vi "createPattern.vi"(7 "Numeric":i32=50, 11 "Refnum in":T1) -> (3 "Image Out 3":T1)   [LabVIEW 2020]
uses:
  <vilib>/vision/Image Controls.llb/IMAQ Image.ctl
  <vilib>/Analysis/1siggen.llb/Ramp Pattern by Samples.vi
  <vilib>/vision/NI_Vision_Development_Module.lvlib
  <vilib>/Analysis/NI_AALBase.lvlib
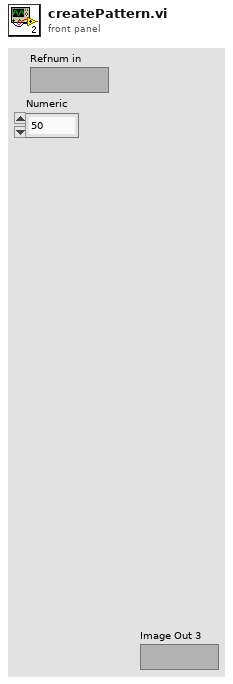
[diagram p1: front panel]
types:
  T1 = typedef "IMAQ Image.ctl" = refnum<image>
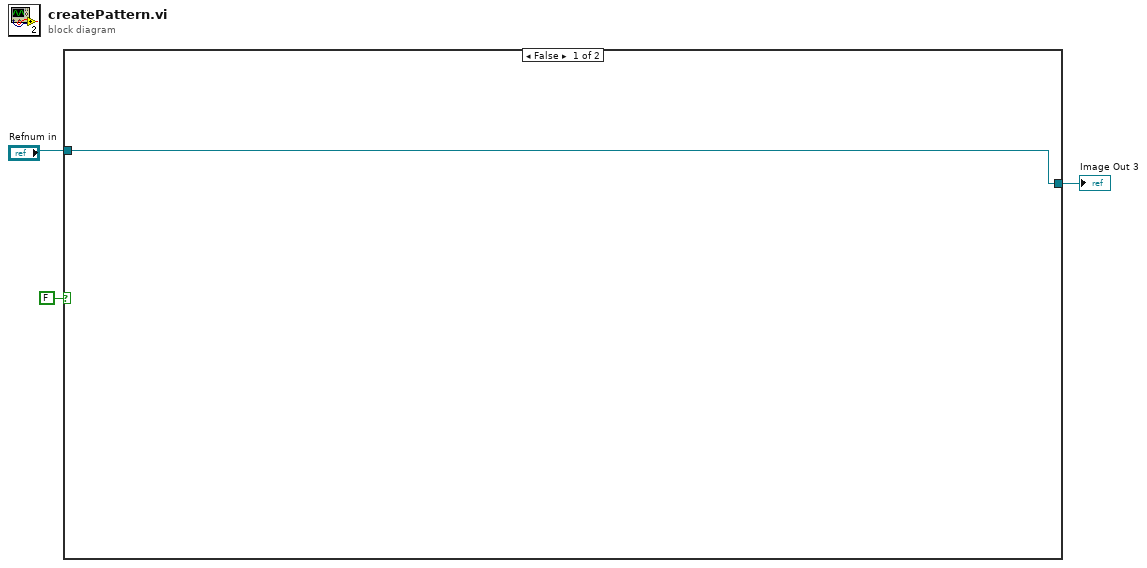
[diagram p0: block diagram]
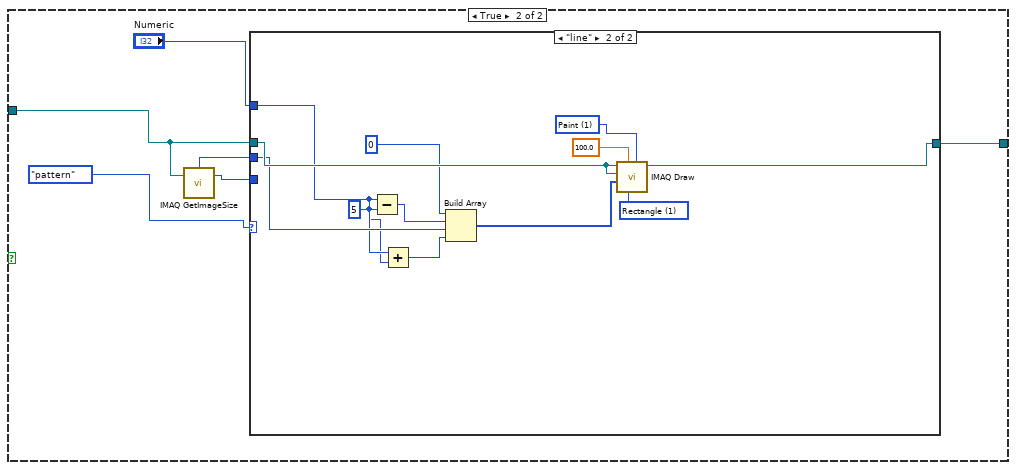
[diagram p2: hidden frame]
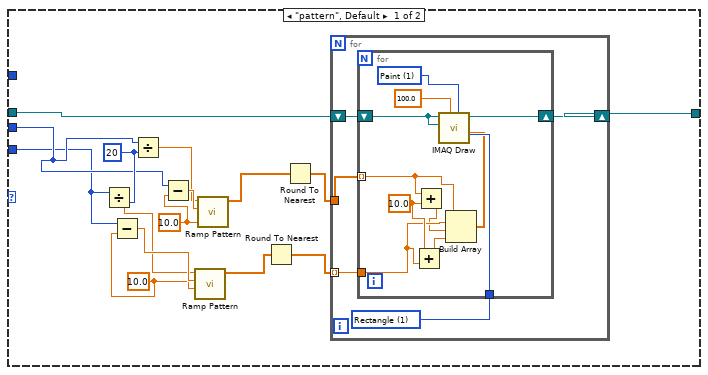
[diagram p3: hidden frame]
diagram:
  n1 = case shown="False" FALSE {
    tunnel: [w4 w10] -> w3
    tunnel: "Refnum in" -> [w4 w5]
    frame False {
    }
    frame True {
      n2 = call "IMAQ GetImageSize"("Image"=w5) -> ("Y Resolution"=w7:i32, "X Resolution"=w8:i32)  [unwired: 3 in, 1 out]
      n3 = case shown="\"line\"" enum16{"pattern", "line"}."pattern" {
        tunnel: w5 -> [w11 w51]
        tunnel: [w14 w50] -> w10
        tunnel: w8 -> [w13 w46]
        tunnel: w7 -> [w12 _]
        tunnel: "Numeric" -> [_ w45]
        frame "pattern", Default {
          w20 = 10.0 ("start")
          w17 = 10.0 ("start")
          w15 = 20 ("y")
          n4 = Divide(x=w12, y=w15) -> (x/y=w19:dbl)
          n5 = Subtract(x=w12, y=w20) -> (x-y=w21:dbl)
          n6 = Divide(x=w13, y=w15) -> (x/y=w16:dbl)
          n7 = Subtract(x=w13, y=w17) -> (x-y=w18:dbl)
          n8 = call-poly <vilib>:"Ramp Pattern.vi"("start"=w20, "end"=w21, "samples"=w19) -> ("Ramp Pattern"=w23:dbl[])  [unwired: 7 in, 1 out]
          n9 = call-poly <vilib>:"Ramp Pattern.vi"("start"=w17, "end"=w18, "samples"=w16) -> ("Ramp Pattern"=w22:dbl[])  [unwired: 7 in, 1 out]
          n10 = Round To Nearest(number=w23) -> (nearest integer value=w25:dbl[])
          n11 = Round To Nearest(number=w22) -> (nearest integer value=w24:dbl[])
          n12 = for {
            shift-right: [w28] -> w14
            shift-left: w11 -> [w29]
            tunnel: w24 -> [w27]
            tunnel: w25 -> [w26] mode=indexing
            w30 = u16 1 items=["Line", "Rectangle", "Oval"] ("Shape to draw")
            n13 = for {
              tunnel: w30 -> [w41]
              tunnel: w27 -> [w35] mode=indexing
              tunnel: w26 -> [w34]
              shift-right: [w37] -> w28
              shift-left: w29 -> [w38]
              w36 = 10.0 ("y")
              w39 = u16 1 items=["Frame", "Paint", "Invert Frame", "Invert Paint"] ("Draw Mode")
              n14 = Add(x=w36, y=w34) -> (x+y=w32:dbl)
              n15 = Add(x=w35, y=w36) -> (x+y=w33:dbl)
              n16 = Build Array(w35, w34, w33, w32) -> (w31:dbl[])
              n17 = call "IMAQ Draw"("Draw Mode"=w39, "Shape to draw"=w41, "Pixel Color"=sgl 100.0, "Coordinates"=w31, "Image Dst"=w38, "Image Src"=w38) -> ("Image Dst Out"=w37:T1)  [unwired: 4 in, 1 out]
            }
          }
        }
        frame "line" {
          w44 = 5 ("y")
          w49 = u16 1 items=["Line", "Rectangle", "Oval"] ("Shape to draw")
          w52 = u16 1 items=["Frame", "Paint", "Invert Frame", "Invert Paint"] ("Draw Mode")
          n18 = Subtract(x=w45, y=w44) -> (x-y=w47:i32)
          n19 = Add(x=w45, y=w44) -> (x+y=w43:i32)
          n20 = Build Array(0, w47, w46, w43) -> (w42:i32[])
          n21 = call "IMAQ Draw"("Draw Mode"=w52, "Shape to draw"=w49, "Pixel Color"=sgl 100.0, "Coordinates"=w42, "Image Dst"=w51, "Image Src"=w51) -> ("Image Dst Out"=w50:T1)  [unwired: 4 in, 1 out]
        }
      }
    }
  }
  "Image Out 3" <- w3
